vi "OpenSfxLib.vi"(6 "Resp Timeout (ms)":i32 min=0, 7 "Enum":T1, 8 "Error In":errorcluster, 10 "RCZ":u16=1 min=1 max=7, 11 "FPGA Reference":refnum<k20>) -> (0 "Error Out":errorcluster, 2 "Open Lib OK":bool, 3 "FPGA VI Reference Out":refnum<k20>)   [LabVIEW 2018]
uses:
  ControlTestSlot.ctl
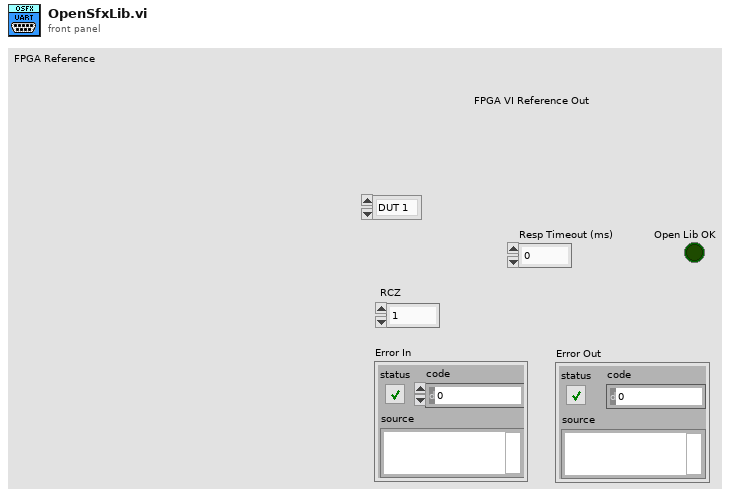
[diagram p1: front panel]
types:
  T1 = typedef "ControlTestSlot.ctl" = enum16{"DUT 1", "DUT 2"}
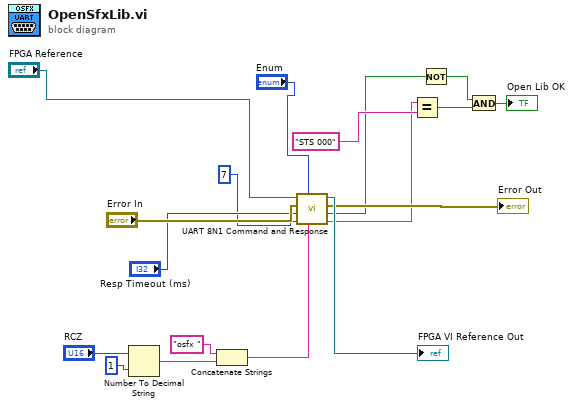
[diagram p0: block diagram]
diagram:
  n1 = Number To Decimal String(number="RCZ", width (-)=i16 1) -> (decimal integer string=w11:string)
  n2 = Concatenate Strings("osfx " ("Text to Send"), w11) -> (w1:string)
  n3 = call "UART 8N1 Command and Response.vi"("Text to Send"=w1, "Active Dut"="Enum", "Response Size (char)"=u32 7, "Response Timeout (ms)"="Resp Timeout (ms)", "Error In"="Error In", "FPGA VI Reference In"="FPGA Reference") -> ("Received Text"=w6:string, "Timeout Flag"=w7:bool, "Error Out"=→"Error Out":errorcluster, "FPGA VI Reference Out"=→"FPGA VI Reference Out":refnum<k20>)  [unwired: 1 in, 1 out]
  n4 = Equal?(x=w6, y="STS 000") -> (x = y?=w16:bool)
  n5 = Not(x=w7) -> (.not. x?=w18:bool)
  n6 = And(x=w18, y=w16) -> (x .and. y?=→"Open Lib OK":bool)
